vi "SetupFullBinning.vi"(8 "error in (no error)":errorcluster) -> (0 "error out":errorcluster)   [LabVIEW 2015, in "ESLSCDLL.lvlib"]
uses:
  ESLSCDLL.lvlib
  Globals.vi
  ESLSCDLL.dll
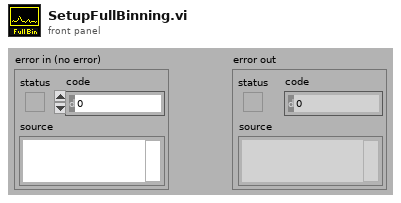
[diagram p1: front panel]
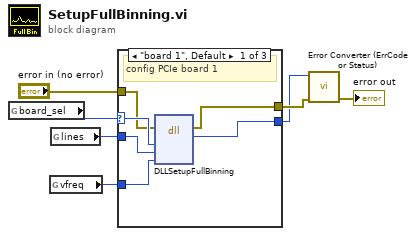
[diagram p0: block diagram]
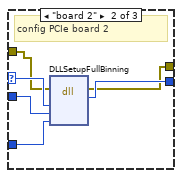
[diagram p2: hidden frame]
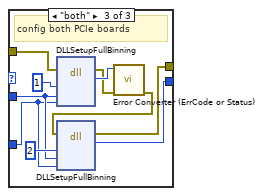
[diagram p3: hidden frame]
diagram:
  n1 = global read "Globals.vi" "board_sel"() -> (w3:enum32{"0", "board 1", "board 2", "both"})
  n2 = global read "Globals.vi" "vfreq"() -> (w1:u32)
  n3 = global read "Globals.vi" "lines"() -> (w2:u32)
  n4 = case shown="\"board 1\", Default" w3 {
    selector: w3 -> [w13 w19 _]
    tunnel: w2 -> [w12 w18 w27]
    tunnel: w1 -> [w11 w17 w26]
    tunnel: "error in (no error)" -> [w10 w14 w25]
    tunnel: [w9 w15 w21] -> w5
    tunnel: [w8 w16 w20] -> w4
    frame "board 1", Default {
      # "config PCIe board 1"
      n5 = dll-call lib="C:/ENTW/PCIE/LV64/board.vis/ESLSCDLL.dll" fn="DLLSetupFullBinning" ("lwlscdll.dll:DLLReadFFLoop")(error in=w10, "drvno"=w13, "lines"=w12, "vfreq"=w11) -> (error out=w9:errorcluster, "es_status_codes"=w8:i32)  [unwired: 5 in, 1 out]
    }
    frame "board 2" {
      # "config PCIe board 2"
      n6 = dll-call lib="C:/ENTW/PCIE/LV64/board.vis/ESLSCDLL.dll" fn="DLLSetupFullBinning" ("lwlscdll.dll:DLLReadFFLoop")(error in=w14, "drvno"=w19, "lines"=w18, "vfreq"=w17) -> (error out=w15:errorcluster, "es_status_codes"=w16:i32)  [unwired: 5 in, 1 out]
    }
    frame "both" {
      # "config both PCIe boards"
      n7 = dll-call lib="C:/ENTW/PCIE/LV64/board.vis/ESLSCDLL.dll" fn="DLLSetupFullBinning" ("lwlscdll.dll:DLLReadFFLoop")(error in=w25, "drvno"=u32 1, "lines"=w27, "vfreq"=w26) -> (error out=w23:errorcluster, "es_status_codes"=w24:i32)  [unwired: 5 in, 1 out]
      n8 = call "Error Converter (ErrCode or Status).vi"("error in (no error)"=w23, "error code"=w24) -> ("error out"=w22:errorcluster)  [unwired: 9 in]
      n9 = dll-call lib="C:/ENTW/PCIE/LV64/board.vis/ESLSCDLL.dll" fn="DLLSetupFullBinning" ("lwlscdll.dll:DLLReadFFLoop")(error in=w22, "drvno"=u32 2, "lines"=w27, "vfreq"=w26) -> (error out=w21:errorcluster, "es_status_codes"=w20:i32)  [unwired: 5 in, 1 out]
    }
  }
  n10 = call "Error Converter (ErrCode or Status).vi"("error in (no error)"=w5, "error code"=w4) -> ("error out"=→"error out":errorcluster)  [unwired: 9 in]
